vi "Main.vi"(8 "error in (no error)":errorcluster, 11 "Process in":refnum<class "FRTS Process.lvclass">) -> (0 "error out":errorcluster, 3 "Process out":refnum<class "FRTS Process.lvclass">)   [LabVIEW 2019, in "TimingDRV Engine.lvlib" / "FRTS Process.lvclass"]
uses:
  FRTS Process.lvclass
  C:/Users/XEnderMD/Desktop/CD Project Tools/Source/Engine/Parent Classes/Process/Process.lvclass
  <vilib>/Platform/TimedLoop/XDataNode/timing_clust.ctl
  <vilib>/Platform/TimedLoop/XDataNode/nitl_modes.ctl
  <vilib>/Platform/TimedLoop/XDataNode/wakeup.ctl
  Parent Classes/Process/Process.lvclass/Process.ctl
  <vilib>/NI VeriStand/Custom Device API/Get Item Property (I32).vi
  Parent Classes/Process/Process.lvclass
  <vilib>/platform/TimedLoop/XDataNode/XDataNode.xnode
  <vilib>/NI VeriStand/Custom Device API/Custom Device API.lvlib
  <vilib>/Platform/TimedLoop/XDataNode/XDNodeRunTimeDep.lvlib
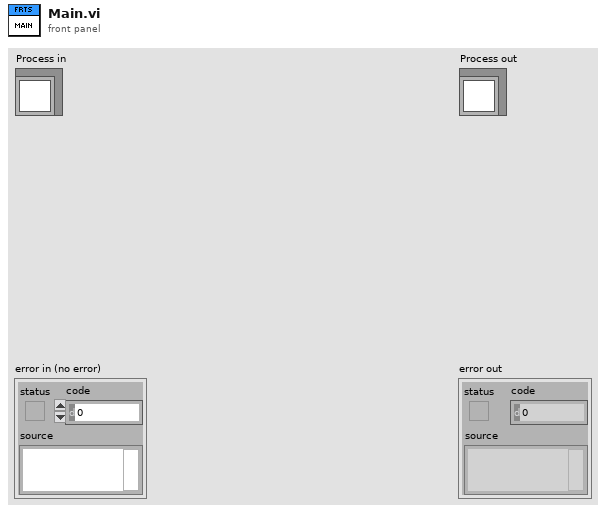
[diagram p1: front panel]
types:
  T1 = typedef "XDNodeRunTimeDep.lvlib/timing_clust.ctl" = cluster{"Expected End [f-1]":u64, "Actual End [f-1]":u64, "Finished Late? [f-1]":bool, "Expected End [i-1]":u64, "Actual End [i-1]":u64, "Finished Late? [i-1]":bool, "Expected Start [i]":u64, "Actual Start [i]":u64, "Expected Start [f]":u64, "Actual Start [f]":u64, "Source Name":string, "Structure Name":string, "Period":i64, "Deadline":i64, "Offset":i64, "Start":i64, "Priority":i32, "Timeout":i32, "Mode":T2, "Wakeup Reason":T3, "Error":errorcluster, "Source Type":string, "Secondary Source Type":string, "Global End Time":u64, "Global Start Time":u64, "Frame Duration":u64, "Iteration Duration":u64, "Assigned CPU":i32, "I/O Scan Engine Mode":u32}
  T2 = typedef "XDNodeRunTimeDep.lvlib/nitl_modes.ctl" = enum32{"No Change", "Process missed periods, maintain original phase", "Discard missed periods, maintain original phase", "Process missed periods, ignore original phase", "Discard missed periods, ignore original phase"}
  T3 = typedef "XDNodeRunTimeDep.lvlib/wakeup.ctl" = enum32{"Normal", "Aborted", "Asynchronous wakeup", "Timing source error", "Timed loop error", "Timeout"}
  T4 = typedef "TimingDRV Engine.lvlib/Process.lvclass/Async Paramters.ctl" = cluster{"Device Reference":T5, "Device Clock":string, "Device Inputs FIFO":refnum<k33>, "Device Outputs FIFO":refnum<k33>, "CD Engine Event Ref":T6}
  T5 = typedef "Custom Device API.lvlib/Custom Device Item Ref.ctl" = u64
  T6 = typedef "Custom Device API.lvlib/Custom Device Engine Event Ref.ctl" = refnum<event-registration>
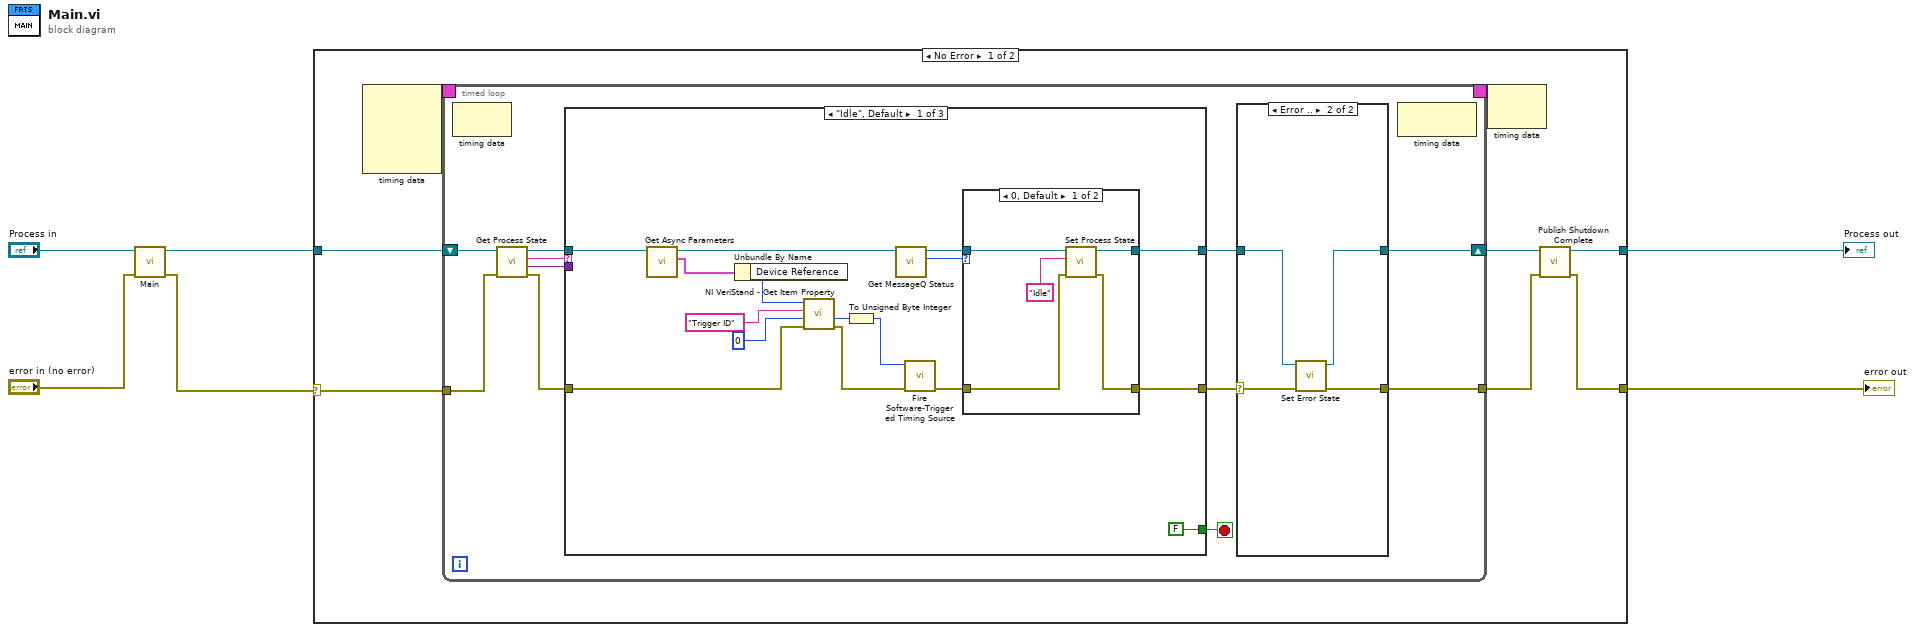
[diagram p0: block diagram]
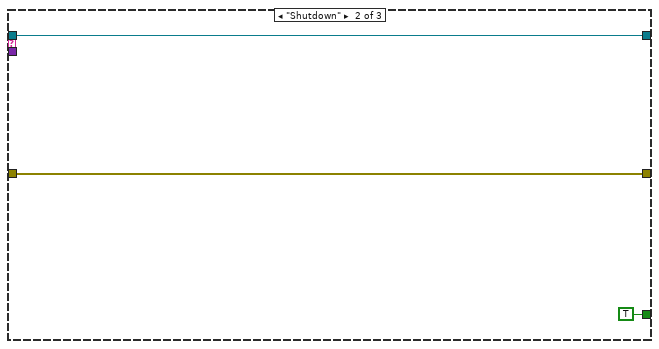
[diagram p4: hidden frame]
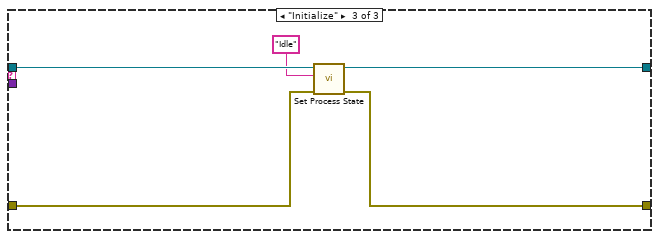
[diagram p5: hidden frame]
diagram:
  n1 = call-parent "Main.vi"("error in (no error)"="error in (no error)", "Process in"="Process in") -> ("error out"=w3:errorcluster, "Process out"=w4:refnum<class "FRTS Process.lvclass">)  [unwired: 8 in]
  n2 = case shown="No Error" w3 {
    selector: w3 -> [w9 w68]
    tunnel: [w11 w68] -> w2
    tunnel: [w13 w67] -> w1
    tunnel: w4 -> [w10 w67]
    frame No Error {
      n3 = node-c288() -> (w8:T1)  [unwired: 4 in]
      n4 = timed-loop {
        shift-right: [w17] -> w14
        shift-left: w10 -> [w24]
        tunnel: w9 -> [w25]
        tunnel: [w16] -> w12
        timing: w8 -> [_]
        timing-out: [_] -> w7
        stop <- w15 stop-if-true
        n5 = node-c288() -> ()  [unwired: 1 in, 1 out]
        n6 = call "Get Process State.vi"("error in (no error)"=w25, "Process in"=w24) -> ("error out"=w20:errorcluster, "Payload"=w21:variant, "Command"=w22:string, "Process out"=w23:refnum<class "FRTS Process.lvclass">)  [unwired: 6 in]
        n7 = case shown="\"Idle\", Default" w22 {
          tunnel: w23 -> [w48 w58 w64]
          tunnel: w21 -> [_ _ _]
          tunnel: w20 -> [w43 w57 w63]
          tunnel: [w37 w58 w62] -> w19
          tunnel: [w36 w57 w61] -> w18
          tunnel: [FALSE TRUE _] -> w15
          frame "Idle", Default {
            n8 = call "Get Async Parameters.vi"("Process in"=w48) -> ("Async Parameters"=w47:T4, "Process out"=w40:refnum<class "FRTS Process.lvclass">)  [unwired: 9 in]
            n9 = Unbundle By Name(w47) -> ("Device Reference"=w42:T5)
            n10 = call-poly <vilib>:"NI VeriStand - Get Item Property.vi"("error in (no error)"=w43, "Default Value"=0, "Property Name"="Trigger ID", "Item Ref in"=w42) -> ("error out"=w41:errorcluster, "Value"=w44:i32)  [unwired: 4 in, 2 out]
            n11 = To Unsigned Byte Integer(number=w44) -> (unsigned 8bit integer=w35:u8)
            n12 = call "Get MessageQ Status.vi"("Process in"=w40) -> ("# elements in MessageQ"=w39:i32, "Process out"=w38:refnum<class "FRTS Process.lvclass">)  [unwired: 7 in, 2 out]
            n13 = call <vilib>:"Fire Software-Triggered Timing Source.vi"("error in (no error)"=w41, "trigger ID"=w35) -> ("error out"=w34:errorcluster)  [unwired: 8 in, 1 out]
            n14 = case shown="0, Default" w39 {
              tunnel: w38 -> [w54 w55]
              tunnel: [w53 w55] -> w37
              tunnel: w34 -> [w52 w56]
              tunnel: [w51 w56] -> w36
              frame 0, Default {
                n15 = call "Set Process State.vi"("error in (no error)"=w52, "Command"="Idle", "Process in"=w54) -> ("error out"=w51:errorcluster, "Process out"=w53:refnum<class "FRTS Process.lvclass">)  [unwired: 7 in]
              }
              frame 1 {
              }
            }
          }
          frame "Shutdown" {
          }
          frame "Initialize" {
            n16 = call "Set Process State.vi"("error in (no error)"=w63, "Command"="Idle", "Process in"=w64) -> ("error out"=w61:errorcluster, "Process out"=w62:refnum<class "FRTS Process.lvclass">)  [unwired: 7 in]
          }
        }
        n17 = case shown="Error .." w18 {
          selector: w18 -> [w28 w33]
          tunnel: w19 -> [w29 w32]
          tunnel: [w29 w31] -> w17
          tunnel: [w28 w30] -> w16
          frame No Error {
          }
          frame Error {
            n18 = call "Set Error State.vi"("error in (no error)"=w33, "Process in"=w32) -> ("error out"=w30:errorcluster, "Process out"=w31:refnum<class "FRTS Process.lvclass">)  [unwired: 8 in]
          }
        }
        n19 = node-c288() -> ()  [unwired: 1 in, 1 out]
      }
      n20 = node-c288(w7) -> ()  [unwired: 1 out]
      n21 = call "Publish Shutdown Complete.vi"("error in (no error)"=w12, "Process in"=w14) -> ("error out"=w11:errorcluster, "Process out"=w13:refnum<class "FRTS Process.lvclass">)  [unwired: 8 in]
    }
    frame Error {
    }
  }
  "error out" <- w2
  "Process out" <- w1
